vi "FaultClearAll.vi"() -> (0 "error out":errorcluster)   [LabVIEW 2015, in "ni-veristand-steps-runtime-lib.lvlib"]
uses:
  ni-veristand-steps-runtime-lib.lvlib
  <vilib>/NI Veristand/Execution/ChannelFaultManager/NI_VS ChannelFault ExecutionAPI.lvlib
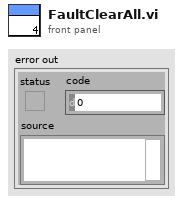
[diagram p1: front panel]
types:
  T1 = typedef "ni-veristand-steps-runtime-lib.lvlib/VeriStand dotNet References.ctl" = cluster{"Project Ref":refnum<k24>, "ModelManager":T2, "AlarmManager":T3, "ChannelFault":T4, "WorkspaceManager":T5}
  T2 = typedef "NI_VS ModelManager ExecutionAPI.lvlib/ModelManagerAPI.ctl" = refnum<k24>
  T3 = typedef "NI_VS AlarmManager ExecutionAPI.lvlib/AlarmManagerAPI.ctl" = refnum<k24>
  T4 = typedef "NI_VS ChannelFault ExecutionAPI.lvlib/ChannelFaultAPI.ctl" = refnum<k24>
  T5 = typedef "NI_VS Workspace ExecutionAPI.lvlib/WorkspaceAPI.ctl" = refnum<k24>
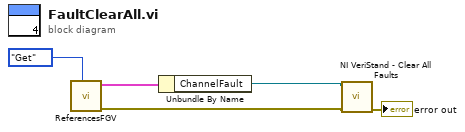
[diagram p0: block diagram]
diagram:
  n1 = call "ReferencesFGV.vi"("Get/Set"=enum16{"Get", "Set"}."Get") -> ("error out"=w2:errorcluster, "VeriStand dotNET Refs out"=w4:T1)  [unwired: 9 in]
  n2 = Unbundle By Name(w4) -> ("ChannelFault"=w3:T4)
  n3 = call <vilib>:"NI VeriStand - Clear All Faults.vi"("error in (no error)"=w2, "ChannelFault in"=w3) -> ("error out"=→"error out":errorcluster)  [unwired: 8 in, 1 out]
